vi "GPS G_StarIV Loop.vi"() -> ()   [LabVIEW 2011]
uses:
  <instrlib>/NavCom SF-2050/NavCom SF-2050.lvlib
panel:
  in  "error in (no error)":errorcluster
  in  "VISA resource name":refnum<visa-resource-name>
  in  "Debug":bool
  in  "Serial Configuration":cluster{"Baud Rate":u32, "Parity":u16}={"Baud Rate"=115200, "Parity"=0} {"Parity" items=["None", "Odd", "Even", "Mark", "Space"]; "Baud Rate" items=["1200"=1200, "2400"=2400, "4800"=4800, "9600"=9600, "19200"=19200, "38400"=38400, "57600"=57600, "115200"=115200]}
  in  "GPS Data Cluster":T1 {"Time"."GPS Time of Week" format="%.3f"; "Velocity, Correction & SET"."Extended Navigation Mode" items=["Non Differential"=0, "Code (RTCM Type 1 & 9)"=1, "Code, Single Frequency (WAAS)"=2, "Code, Dual Frequency (WAAS)"=3, "Code, Single Frequency (WCT)"=4, "Code/RCP, Dual Frequency (WCT)"=5, "Code, Single Frequency (RTG)"=6, "Code (RTCM Type 1 & 9) Dual Frequency"=10, "Code/RCP, Dual Frequency (RTG)"=11, "Code, Single Frequency (NCT-RTK)"=12, "Code, Single Frequency (RTCM 18 & 19)"=13, "Code, Single Frequency (RTCM 21 & 22)"=14, "Code, Single Frequency (CMR)"=15, "Code, Dual Frequency (NCT-RTK)"=16, "Code, Dual Frequency (RTCM 18 & 19)"=17, "Code, Dual Frequency (RTCM 20 & 21)"=18, "Code, Dual Frequency (CMR)"=19, "RTK (NCT-RTK)"=20, "RTK (RTCM 18 & 19)"=21, "RTK (RTCM 20 & 21)"=22, "RTK (CMR)"=23, "Code, Single Frequency with SET (RTG)"=24, "Code/RCP, Dual Frequency with SET (RTG)"=25, "RTK Extend"=26]}
  out "GPS Data":T1 {"Time"."GPS Time of Week" format="%.3f"; "Velocity, Correction & SET"."Extended Navigation Mode" items=["Non Differential"=0, "Code (RTCM Type 1 & 9)"=1, "Code, Single Frequency (WAAS)"=2, "Code, Dual Frequency (WAAS)"=3, "Code, Single Frequency (WCT)"=4, "Code/RCP, Dual Frequency (WCT)"=5, "Code, Single Frequency (RTG)"=6, "Code (RTCM Type 1 & 9) Dual Frequency"=10, "Code/RCP, Dual Frequency (RTG)"=11, "Code, Single Frequency (NCT-RTK)"=12, "Code, Single Frequency (RTCM 18 & 19)"=13, "Code, Single Frequency (RTCM 21 & 22)"=14, "Code, Single Frequency (CMR)"=15, "Code, Dual Frequency (NCT-RTK)"=16, "Code, Dual Frequency (RTCM 18 & 19)"=17, "Code, Dual Frequency (RTCM 20 & 21)"=18, "Code, Dual Frequency (CMR)"=19, "RTK (NCT-RTK)"=20, "RTK (RTCM 18 & 19)"=21, "RTK (RTCM 20 & 21)"=22, "RTK (CMR)"=23, "Code, Single Frequency with SET (RTG)"=24, "Code/RCP, Dual Frequency with SET (RTG)"=25, "RTK Extend"=26]; "Altitude" format="%#_18g"; "Longitude" format="%#_18g"; "Latitude" format="%#_18g"}
  out "error out":errorcluster
  in  "stop?":bool
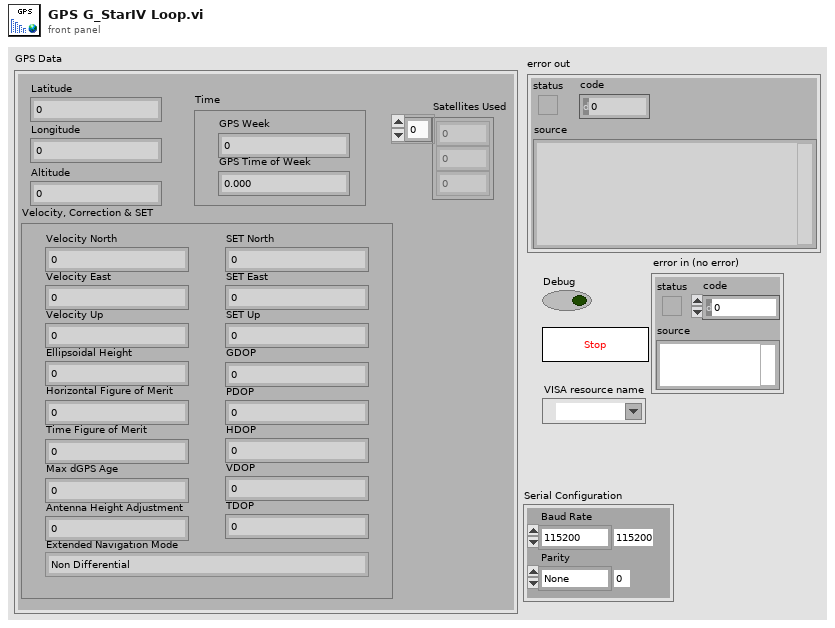
[diagram p1: front panel]
types:
  T1 = cluster{"Latitude":dbl, "Longitude":dbl, "Altitude":dbl, "Velocity, Correction & SET":cluster{"Velocity North":dbl, "Velocity East":dbl, "Velocity Up":dbl, "Ellipsoidal Height":dbl, "GDOP":sgl, "PDOP":sgl, "HDOP":sgl, "VDOP":sgl, "TDOP":sgl, "Horizontal Figure of Merit":u8, "Time Figure of Merit":u8, "Max dGPS Age":sgl, "Extended Navigation Mode":u8, "Antenna Height Adjustment ":dbl, "SET North":i32, "SET East":i32, "SET Up":i32}, "Time":cluster{"GPS Week":u16, "GPS Time of Week":sgl}, "Satellites Used":i32[]}
  T2 = cluster{"Velocity North":dbl, "Velocity East":dbl, "Velocity Up":dbl, "Ellipsoidal Height":dbl, "GDOP":sgl, "PDOP":sgl, "HDOP":sgl, "VDOP":sgl, "TDOP":sgl, "Horizontal Figure of Merit":u8, "Time Figure of Merit":u8, "Max dGPS Age":sgl, "Extended Navigation Mode":u8, "Antenna Height Adjustment ":dbl, "SET North":i32, "SET East":i32, "SET Up":i32}
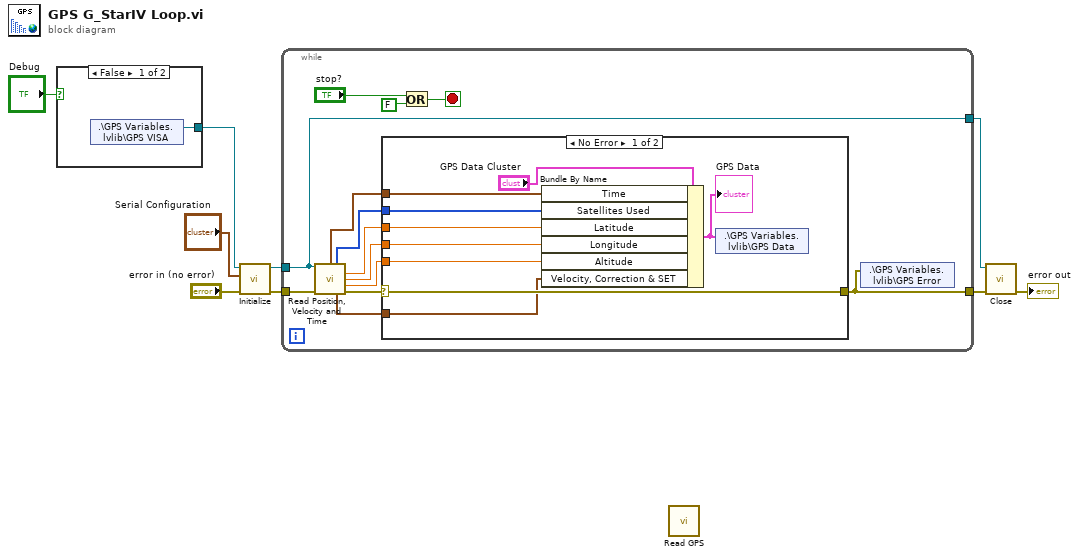
[diagram p0: block diagram]
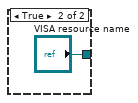
[diagram p3: hidden frame]
diagram:
  n1 = case shown="False" "Debug" {
    tunnel: [w10 "VISA resource name"] -> w4
    frame False {
      n2 = shared-variable ".\\GPS Variables.lvlib\\GPS VISA"() -> (w10:refnum<visa-resource-name>)  [unwired: 1 in, 1 out]
    }
    frame True {
    }
  }
  n3 = call <instrlib>:"Initialize.vi"("error in (no error)"="error in (no error)", "Serial Configuration"="Serial Configuration", "VISA resource name"=w4) -> ("error out"=w2:errorcluster, "VISA resource name out"=w1:refnum<visa-resource-name>)  [unwired: 7 in]
  n4 = while {
    tunnel: w1 -> [w22]
    tunnel: w2 -> [w23]
    tunnel: [w22] -> w9
    tunnel: [w12] -> w8
    stop <- w20 stop-if-true
    n5 = call <instrlib>:"Read Position, Velocity and Time.vi"("VISA resource name"=w22, "error in (no error)"=w23) -> ("Time"=w14:cluster{"GPS Week":u16, "GPS Time of Week":sgl}, "Satellites Used"=w15:i32[], "Latitude"=w19:dbl, "Longitude"=w18:dbl, "Altitude"=w17:dbl, "Velocity, Correction & SET"=w16:T2, "error out"=w21:errorcluster)  [unwired: 6 in, 1 out]
    n6 = case shown="No Error" w21 {
      selector: w21 -> [w33 w34]
      tunnel: [w33 w34] -> w12
      tunnel: w19 -> [w32 _]
      tunnel: w18 -> [w31 _]
      tunnel: w17 -> [w30 _]
      tunnel: w16 -> [w29 _]
      tunnel: w15 -> [w28 _]
      tunnel: w14 -> [w27 _]
      frame No Error {
        n7 = Bundle By Name(cluster="GPS Data Cluster", "Time"=w27, "Satellites Used"=w28, "Latitude"=w32, "Longitude"=w31, "Altitude"=w30, "Velocity, Correction & SET"=w29) -> (w26:T1)
        "GPS Data" <- w26
        n8 = shared-variable ".\\GPS Variables.lvlib\\GPS Data"(w26) -> ()  [unwired: 1 in, 1 out]
      }
      frame Error {
      }
    }
    n9 = Or(x="stop?", y=FALSE) -> (x .or. y?=w20:bool)
    n10 = shared-variable ".\\GPS Variables.lvlib\\GPS Error"(w12) -> ()  [unwired: 1 in, 1 out]
  }
  n11 = call "Read GPS.vi"() -> ()  [unwired: 12 in, 4 out]
  n12 = call <instrlib>:"Close.vi"("error in (no error)"=w8, "VISA resource name"=w9) -> ("error out"=→"error out":errorcluster)  [unwired: 9 in]
